vi "Read a tag from DAQ Test Program.vi"() -> ()   [LabVIEW 2018, in "DAQ.lvlib"]
uses:
  DAQ.lvlib
  Tag VIs/Tag FGV Operation Enum.ctl
  Shared Variables/Dynamic Shared Variables.lvlib
panel:
  out "error out":errorcluster
  in  "error in (no error)":errorcluster
  out "Variant":variant
  out "Input Channel Tag Name":string
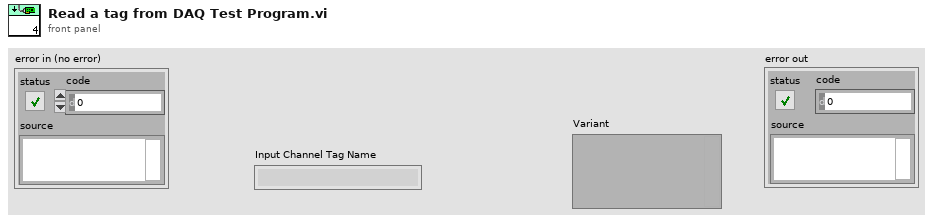
[diagram p1: front panel]
types:
  T1 = typedef "Tag FGV Operation Enum.ctl" = enum16{"Init", "Set Notification Queue", "Create Tag", "Commit", "Write Tag (Numeric)", "Write Tag (Boolean)", "Read All Tags", "Read One Tag", "Delete Tag Category", "Set Alarm Parameters (Numeric)", "Set Alarm Parameters (Boolean)", "Enable All Alarms", "Disable All Alarms", "Delete All Tags", "Read Alarms", "Ack Alarm", "Read Alarm Parameters (Numeric)", "Read Alarm Parameters (Boolean)"}
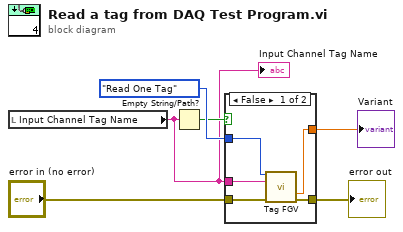
[diagram p0: block diagram]
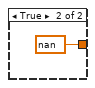
[diagram p2: hidden frame]
diagram:
  n1 = local read "Input Channel Tag Name"() -> (w3:string)
  "Input Channel Tag Name" <- w3
  n2 = Empty String/Path?(string/path=w3) -> (empty?=w5:bool)
  n3 = case shown="False" w5 {
    tunnel: Tag_FGV_Operation_Enum."Read One Tag" ("Operation") -> [w11 _]
    tunnel: [w10 nan ("Tag Value")] -> w4
    tunnel: [w9 _] -> w1
    tunnel: w3 -> [w8 _]
    tunnel: "error in (no error)" -> [w7 _]
    frame False {
      n4 = call "Tag FGV.vi"("Operation"=w11, "Tag Name"=w8, "error in (no error)"=w7) -> ("Tag Value"=w10:dbl, "error out"=w9:errorcluster)  [unwired: 5 in, 6 out]
    }
    frame True {
    }
  }
  "Variant" <- w4
  "error out" <- w1
